vi "PCO_SetIRSensitivity.vi"(8 "error in (no error)":errorcluster {"code" format="%x"}, 10 "wIR":u16(ring) items=["OFF", "ON"], 11 "ph":u64) -> (0 "error out":errorcluster {"code" format="%x"}, 2 "ErrorMessage":i32 format="%x", 3 "ph out":u64)   [LabVIEW 2019, in "SDK.lvlib" / "ImageSensor.lvlib"]
doc: "<b>Description:</b>\nThis function does set the IR sensitivity operating mode. This option is only available for special camera models with image sensors that have improved IR sensitivity. Availability of this option can be checked with the parameter wIRDESC of the PCO_Description structure. If IR sensitivity is activated limits for the delay and exposure times are defined through parameters dwMinDelayIRDESC, dwMaxDelayIRDESC, dwMinExposIRDESC and dwMaxExposIRDESC of the PCO_Description structure.\n\n<b>Supported camera type:</b>\npco.pixelfly_usb, pco.1300, pco.1400\n\n<b>Descriptor dependency:</b>\nwIRDESC"
uses:
  ImageSensor.lvlib
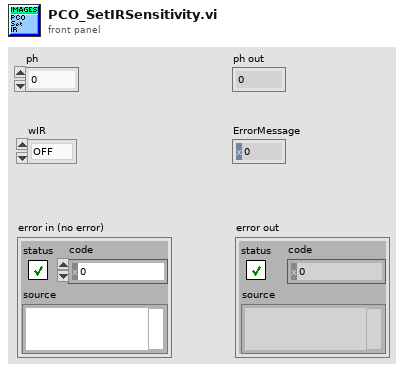
[diagram p1: front panel]
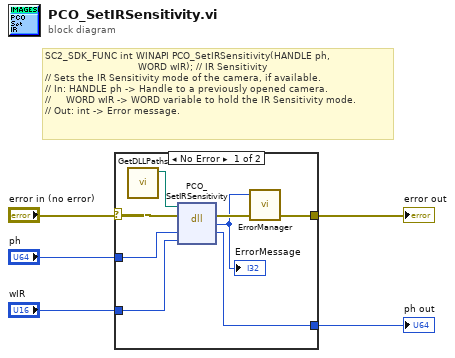
[diagram p0: block diagram]
diagram:
  # "SC2_SDK_FUNC int WINAPI PCO_SetIRSensitivity(HANDLE ph,\n                               WORD wIR); // IR Sensitivity\n// Sets the IR Sensitivity mode of the camera, if available.\n// In: HANDLE ph -> Handle to a previously opened camera.\n//     WORD wIR -> WORD variable to hold the IR Sensitivity mode.\n// Out: int -> Error message."
  n1 = case shown="No Error" "error in (no error)" {
    selector: "error in (no error)" -> [w10 w15]
    tunnel: "ph" -> [w13 w14]
    tunnel: [w12 w14] -> w4
    tunnel: "wIR" -> [w11 _]
    tunnel: [w8 w15] -> w2
    frame No Error {
      n2 = call "GetDLLPaths.vi"() -> ("SC2_Cam_Path"=w6:path)  [unwired: 8 in, 3 out]
      n3 = dll-call lib="?" fn="PCO_SetIRSensitivity"(path in=w6, error in=w10, "ph"=w13, "wIR"=w11) -> (error out=w9:errorcluster, "return type"=w7:i32, "ph"=w12:u64)  [unwired: 2 in, 1 out]
      "ErrorMessage" <- w7
      n4 = call "ErrorManager.vi"("error in (no error)"=w9, "error code"=w7) -> ("error out"=w8:errorcluster)  [unwired: 2 in, 1 out]
    }
    frame Error {
    }
  }
  "ph out" <- w4
  "error out" <- w2
